vi "LJUD UE9RAW EraseMem.vi"(7 "Comm Settings":T1={"Open LabJack "=TRUE, "Use USB"=TRUE, "IP Address"="192.168.1.209", "PortA"=52360, "PortB"=0}, 8 "error in (no error)":errorcluster, 9 "Key":u8 format="%.0x", 10 "EraseArea":u8 format="%.0x", 11 "Handle In":i32) -> (0 "error out":errorcluster, 3 "Handle Out":i32)   [LabVIEW 2021]
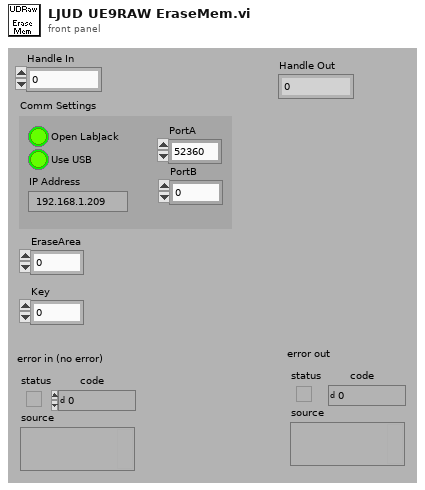
[diagram p1: front panel]
types:
  T1 = cluster{"Open LabJack ":bool, "Use USB":bool, "IP Address":string, "PortA":u16, "PortB":u16}
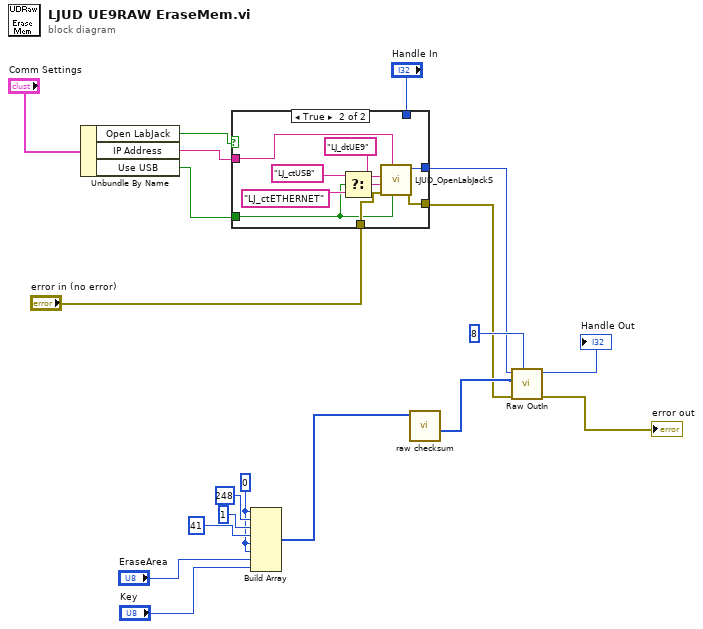
[diagram p0: block diagram]
diagram:
  w15 = u8 0 ("Input Element")
  n1 = Unbundle By Name("Comm Settings") -> ("Open LabJack"=w7:bool, "IP Address"=w6:string, "Use USB"=w5:bool)
  n2 = case shown="True" w7 {
    tunnel: w6 -> [_ w24]
    tunnel: "error in (no error)" -> [w21 w28]
    tunnel: [w21 w27] -> w3
    tunnel: [w20 w25] -> w2
    tunnel: w5 -> [_ w26]
    tunnel: "Handle In" -> [w20 _]
    frame False {
    }
    frame True {
      n3 = Select(t="LJ_ctUSB" ("ConnectionType"), s=w26, f="LJ_ctETHERNET" ("ConnectionType")) -> (s? t:f=w22:string)
      n4 = call "LJUD_OpenLabJackS.vi"("FirstFound"=w26, "Address"=w24, "error in"=w28, "ConnectionType"=w22, "DeviceType"="LJ_dtUE9") -> ("error out"=w27:errorcluster, "Handle"=w25:i32)  [unwired: 4 in, 1 out]
    }
  }
  n5 = Build Array(w15, u8 248 ("Input Element"), u8 1 ("Input Element"), u8 41 ("Input Element"), w15, w15, "EraseArea", "Key") -> (w16:u8[])
  n6 = call "raw checksum.vi"("Array"=w16) -> ("Array Output"=w13:u8[])  [unwired: 3 in, 7 out]
  n7 = call "Raw OutIn.vi"("# of bytes to read in"=8 ("# of bytes to read"), "error in"=w3, "Raw Out"=w13, "Handle In"=w2) -> ("error out"=→"error out":errorcluster, "Handle Out"=→"Handle Out":i32)  [unwired: 4 in, 2 out]
